vi "SSC Digital Calculate Per-Instrument to Per-Site LUT.vi"(0 "Digital SSC In":T2[](array[typedef]), 7 "Sites":i32[](array[numeric])) -> (4 "Per-Instrument to Per-Site LUT":T1[](array[typedef]))   [LabVIEW 2020]
uses:
  SSC Digital/SSC Digital.ctl
  Digital 1D Location Array in a Cluster.ctl
  Shared SubVIs/Trim Whitespace [Inlined].vi
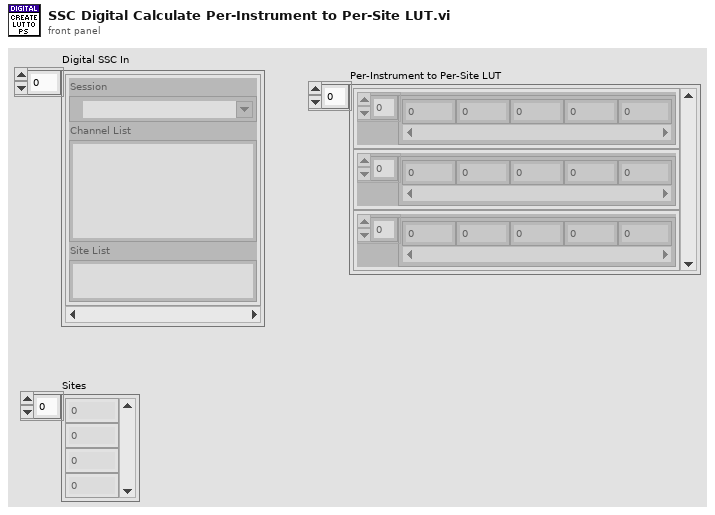
[diagram p1: front panel]
types:
  T1 = typedef "Digital 1D Location Array in a Cluster.ctl" = cluster{"Digital 1D Location Array":i32[]}
  T2 = typedef "SSC Digital.ctl" = cluster{"Session":refnum<k15>, "Channel List":string, "Site List":string}
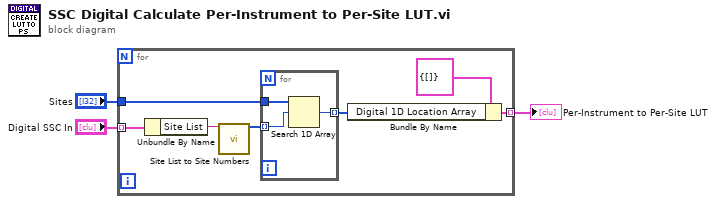
[diagram p0: block diagram]
diagram:
  n1 = for {
    tunnel: "Digital SSC In" -> [w10] mode=indexing
    tunnel: "Sites" -> [w9]
    tunnel: [w7] -> w1 mode=indexing
    n2 = Unbundle By Name(w10) -> ("Site List"=w6:string)
    n3 = call "Site List to Site Numbers.vi"("Site List"=w6) -> ("Site Numbers"=w5:i32[])  [unwired: 13 in, 1 out]
    n4 = for {
      tunnel: w5 -> [w12] mode=indexing
      tunnel: w9 -> [w13]
      tunnel: [w11] -> w8 mode=indexing
      n5 = Search 1D Array(1D array=w13, element=w12) -> (index of element=w11:i32)  [unwired: 1 in]
    }
    n6 = Bundle By Name(cluster=T1 {"Digital 1D Location Array"=[]} ("Digital 1D Location Array in a Cluster"), "Digital 1D Location Array"=w8) -> (w7:T1)
  }
  "Per-Instrument to Per-Site LUT" <- w1
